vi "Pump Status.vi"(8 "error in (no error)":errorcluster, 11 "VICI Settings In":T1) -> (0 "error out":errorcluster, 1 "Connection Error":bool, 2 "Pump On?":enum16{"Off", "On", "Not Initialized"}(ring), 3 "VICI Settings Out":T1)   [LabVIEW 2018, in "VICI M6 M50 Party Mode.lvlib"]
uses:
  VICI M6 M50 Party Mode.lvlib
  Settings Cluster.ctl
  <vilib>/Instr/_visa.llb/VISA Flush IO Buffer Mask.ctl
  VICI Global Library.lvlib
  <vilib>/Instr/_visa.llb/VISA Configure Serial Port (Instr).vi
panel:
  out "read buffer 4":string
  out "read buffer 3":string
  out "read buffer 2":string
  out "number of replacements 2":i32
  out "concatenated string":string
  out "number of replacements":i32
  out "result string":string
  out "read buffer":string
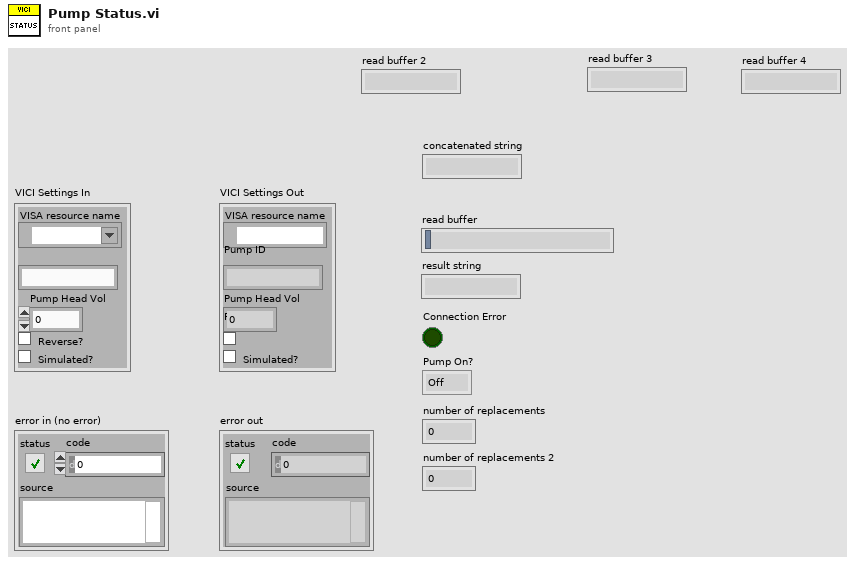
[diagram p1: front panel]
types:
  T1 = typedef "VICI M6 M50 Party Mode.lvlib/Settings Cluster.ctl" = cluster{"VISA resource name":refnum<visa-resource-name>, "Pump ID":string, "Pump Head Vol":dbl, "Reverse?":bool, "Simulated?":bool}
  T2 = typedef "VISA Flush IO Buffer Mask.ctl" = u16
  T3 = typedef "VICI M6 M50 Party Mode.lvlib/VICI Global Library.lvlib/VICI Global.ctl" = cluster{"Busy":bool, "VISA #":string, "Current Pump":string, "Current Function":string, "Pump Array":string[], "Last Success":timestamp, "ID Queue":string[]}
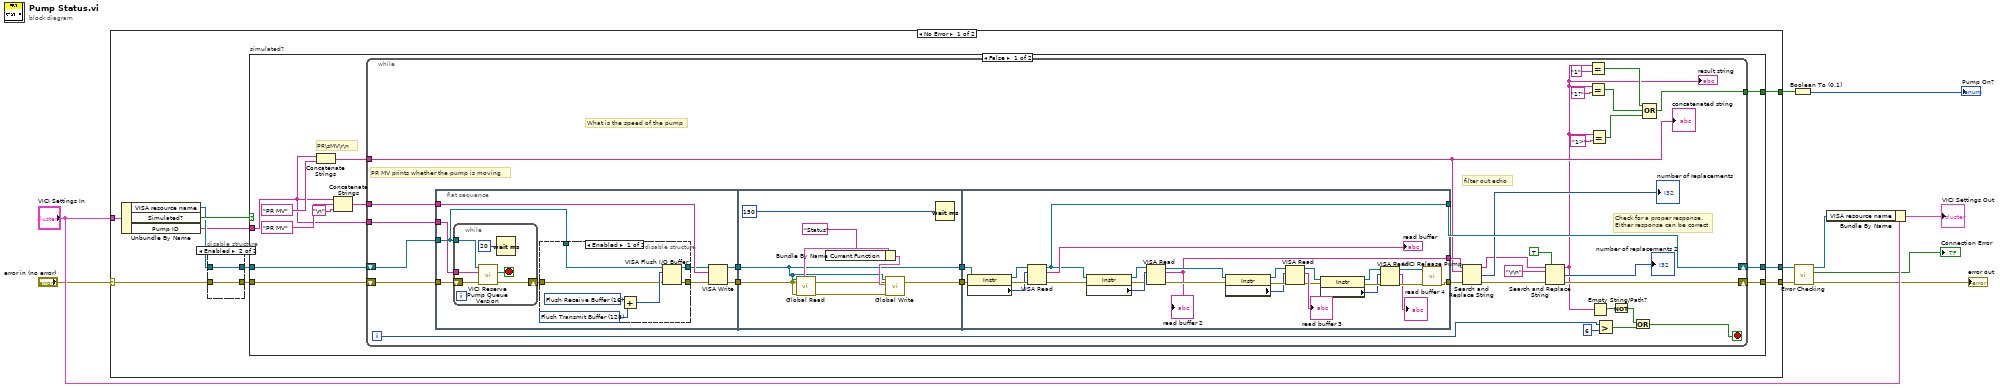
[diagram p0: block diagram]
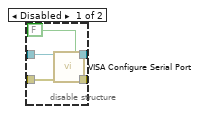
[diagram p2: hidden frame]
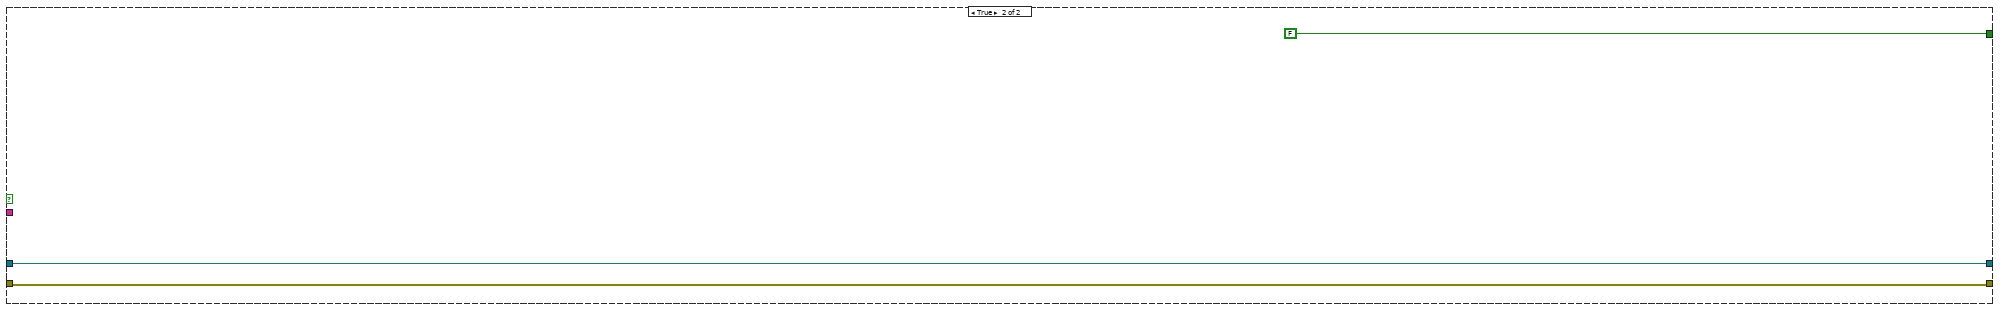
[diagram p4: hidden frame]
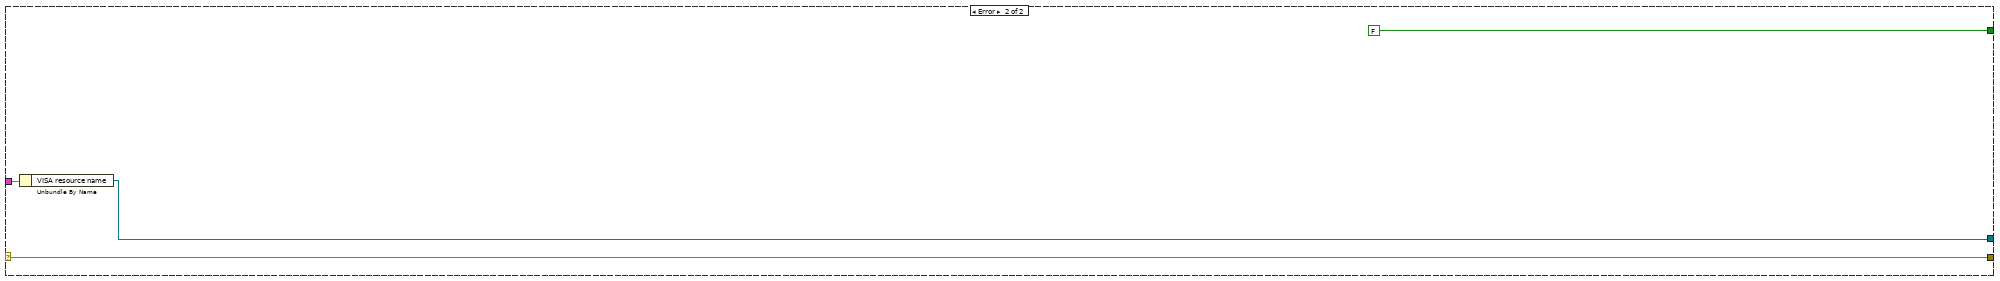
[diagram p5: hidden frame]
diagram:
  n1 = case shown="No Error" "error in (no error)" {
    selector: "error in (no error)" -> [w14 w136]
    tunnel: [w20 w136] -> w8
    tunnel: "VICI Settings In" -> [w19 w135]
    tunnel: [w18 w134] -> w5
    tunnel: [w12 FALSE] -> w2
    frame No Error {
      n2 = Unbundle By Name(w19) -> ("VISA resource name"=w16:refnum<visa-resource-name>, "Simulated?"=w17:bool, "Pump ID"=w11:string)
      n3 = disable-structure shown="Enabled" {
        disable-tunnel: w16 -> [w25 w27]
        disable-tunnel: [w24 w27] -> w15
        disable-tunnel: w14 -> [w22 w26]
        disable-tunnel: [w21 w26] -> w13
        frame Disabled {
          n4 = call-poly "VISA Configure Serial Port"("VISA resource name"=w25, "Enable Termination\nChar (T)"=FALSE ("Enable Termination\nChar (T)"), "error in (no error)"=w22) -> ("VISA resource name out"=w24:refnum<visa-resource-name>, "error out"=w21:errorcluster)  [unwired: 11 in]
        }
        frame Enabled {
        }
      }
      n5 = case "simulated?" shown="False" w17 {
        tunnel: [w31 w132] -> w20
        tunnel: [w38 w130] -> w18
        tunnel: w13 -> [w32 w132]
        tunnel: w15 -> [w29 w130]
        tunnel: [w28 FALSE] -> w12
        tunnel: w11 -> [w30 _]
        frame False {
          # "PR\\sMV\\r\\n"
          n6 = Concatenate Strings(w30, "PR MV" ("search string")) -> (w33:string)
          n7 = Concatenate Strings(w30, "PR MV" ("string"), "\n") -> (w35:string)
          n8 = while {
            tunnel: w35 -> [w63]
            tunnel: w33 -> [w62]
            tunnel: w30 -> [w52]
            tunnel: [w47] -> w28
            shift-right: [w54] -> w31
            shift-left: w32 -> [w60]
            shift-right: [w67] -> w38
            shift-left: w29 -> [w51]
            i -> [w43]
            stop <- w42 stop-if-true
            # "What is the speed of the pump"
            # "filter out echo"
            # "Check for a proper response. \nEither response can be correct"
            # "PR MV prints whether the pump is moving"
            n9 = flat-sequence {
              tunnel: [w79] -> w71
              tunnel: [w80] -> w70
              tunnel: w63 -> [w78]
              tunnel: w51 -> [w75]
              tunnel: w60 -> [w77]
              tunnel: w52 -> [w76]
              tunnel: w71 -> [w97]
              tunnel: w70 -> [w96]
              tunnel: [w96] -> w69
              tunnel: [w97] -> w68
              tunnel: w69 -> [w129]
              tunnel: w68 -> [w128]
              tunnel: [w103] -> w66
              tunnel: [w123] -> w65
              tunnel: [w119] -> w67
              frame #0 {
                n10 = while {
                  tunnel: w75 -> [w93]
                  tunnel: w76 -> [w90]
                  shift-right: [w91] -> w73
                  shift-left: w77 -> [w94]
                  stop <- w92 stop-if-true
                  n11 = call "VICI Reserve Pump Queue Version.vi"("error in (no error)"=w94, "Pump ID"=w90, "VISA # in"=w93) -> ("error out"=w91:errorcluster, "Loop Completed"=w92:bool)  [unwired: 6 in, 1 out]
                  n12 = Wait (ms)(milliseconds to wait=u32 20) -> ()  [unwired: 1 out]
                }
                n13 = disable-structure shown="Enabled" {
                  disable-tunnel: w75 -> [w84 w89]
                  disable-tunnel: [w83 w89] -> w74
                  disable-tunnel: w73 -> [w82 w88]
                  disable-tunnel: [w81 w88] -> w72
                  frame Enabled {
                    w86 = T2 128 items=["Flush Receive Buffer"=16, "Write Transmit Buffer to Device"=32, "Flush Receive Buffer (No I/O)"=64, "Flush Transmit Buffer"=128] ("Mask")
                    w87 = T2 16 items=["Flush Receive Buffer"=16, "Write Transmit Buffer to Device"=32, "Flush Receive Buffer (No I/O)"=64, "Flush Transmit Buffer"=128] ("Mask")
                    n14 = Add(x=w87, y=w86) -> (x+y=w85:T2)
                    n15 = VISA Flush I/O Buffer(VISA resource name=w84, mask (16)=w85, error in (no error)=w82) -> (VISA resource name out=w83:refnum<visa-resource-name>, error out=w81:errorcluster)
                  }
                  frame Disabled {
                  }
                }
                n16 = VISA Write(VISA resource name=w74, write buffer=w78, error in (no error)=w72) -> (VISA resource name out=w79:refnum<visa-resource-name>, error out=w80:errorcluster)  [unwired: 1 out]
              }
              frame #1 {
                n17 = call "Global Read.vi"("VISA #"=w97, "error in (no error)"=w96) -> ("Global for this VISA"=w100:T3, "error out"=w101:errorcluster)  [unwired: 2 in, 5 out]
                n18 = Bundle By Name(cluster=w100, "Current Function"="Status") -> (w99:T3)
                n19 = call "Global Write.vi"("error in (no error)"=w101, "VICI Global"=w99, "VISA # in"=w97) -> ()  [unwired: 7 in, 2 out]
                n20 = Wait (ms)(milliseconds to wait=u32 150) -> ()  [unwired: 1 out]
              }
              frame #2 {
                n21 = property class="Instr"(reference=w128, error in=w129) -> (reference out=w127:refnum<visa-resource-name>, error out=w126:errorcluster, "Serial Settings:Number of Bytes at Serial Port"=w125:u32)
                n22 = VISA Read(VISA resource name=w127, byte count=w125, error in (no error)=w126) -> (VISA resource name out=w119:refnum<visa-resource-name>, read buffer=→"read buffer":string, error out=w118:errorcluster)  [unwired: 1 out]
                n23 = property class="Instr"(reference=w119, error in=w118) -> (reference out=w120:refnum<visa-resource-name>, error out=w121:errorcluster, "Serial Settings:Number of Bytes at Serial Port"=w122:u32)
                n24 = VISA Read(VISA resource name=w120, byte count=w122, error in (no error)=w121) -> (VISA resource name out=w107:refnum<visa-resource-name>, read buffer=w103:string, error out=w115:errorcluster)  [unwired: 1 out]
                "read buffer 2" <- w103
                n25 = property class="Instr"(reference=w107, error in=w115) -> (reference out=w106:refnum<visa-resource-name>, error out=w117:errorcluster, "Serial Settings:Number of Bytes at Serial Port"=w116:u32)
                n26 = VISA Read(VISA resource name=w106, byte count=w116, error in (no error)=w117) -> (VISA resource name out=w105:refnum<visa-resource-name>, read buffer=→"read buffer 3":string, error out=w113:errorcluster)  [unwired: 1 out]
                n27 = property class="Instr"(reference=w105, error in=w113) -> (reference out=w104:refnum<visa-resource-name>, error out=w112:errorcluster, "Serial Settings:Number of Bytes at Serial Port"=w109:u32)
                n28 = VISA Read(VISA resource name=w104, byte count=w109, error in (no error)=w112) -> (VISA resource name out=w110:refnum<visa-resource-name>, read buffer=→"read buffer 4":string, error out=w111:errorcluster)  [unwired: 1 out]
                n29 = call "VICI Release Pump.vi"("error in (no error)"=w111, "VISA # in"=w110) -> ("error out"=w123:errorcluster)  [unwired: 8 in, 1 out]
              }
            }
            n30 = Search and Replace String(input string=w66, search string=w62, error in=w65) -> (result string=w57:string, number of replacements=→"number of replacements":i32, error out=w55:errorcluster)  [unwired: 5 in, 1 out]
            n31 = Search and Replace String(replace all?=TRUE ("replace all? (F)"), input string=w57, search string="\r\n", error in=w55) -> (result string=w41:string, number of replacements=→"number of replacements 2":i32, error out=w54:errorcluster)  [unwired: 4 in, 1 out]
            "result string" <- w41
            n32 = Equal?(x=w41, y="1") -> (x = y?=w50:bool)
            n33 = Equal?(x=w41, y="1?") -> (x = y?=w49:bool)
            n34 = Equal?(x=w41, y="1>") -> (x = y?=w48:bool)
            n35 = Empty String/Path?(string/path=w41) -> (empty?=w39:bool)
            n36 = Greater?(x=w43, y=6) -> (0:w44:bool)
            n37 = Not(x=w39) -> (.not. x?=w40:bool)
            n38 = Or(x=w40, y=w44) -> (x .or. y?=w42:bool)
            n39 = Compound Arithmetic op=OR(w50, w49, w48) -> (w47:bool)
            "concatenated string" <- w62
          }
        }
        frame True {
        }
      }
    }
    frame Error {
      n40 = Unbundle By Name(w135) -> ("VISA resource name"=w134:refnum<visa-resource-name>)
    }
  }
  n41 = Boolean To (0,1)(Boolean=w2) -> (0, 1=→"Pump On?":i16)
  n42 = call "Error Checking.vi"("error in (no error)"=w8, "VISA resource name"=w5) -> ("error out"=→"error out":errorcluster, "Connection Error"=→"Connection Error":bool, "VISA resource name"=w4:refnum<visa-resource-name>)  [unwired: 7 in]
  n43 = Bundle By Name(cluster="VICI Settings In", "VISA resource name"=w4) -> (→"VICI Settings Out":T1)
